vi "optimum.vi"() -> ()   [LabVIEW 2020]
uses:
  <vilib>/MakerHub/LINX/Public/Peripherals/Digital/Digital Read 1 Chan.vi
  <vilib>/MakerHub/LINX/Public/Peripherals/PWM/PWM Set Duty Cycle 1 Chan.vi
  <vilib>/MakerHub/LINX/Public/Peripherals/Digital/Digital Read N Chans.vi
  <vilib>/MakerHub/LINX/Private/Local IO/LinxDigitalRead.vi
  <vilib>/MakerHub/LINX/Public/Utilities/Check Channel.vi
  <vilib>/MakerHub/LINX/Public/Utilities/Open Serial.vi
  <vilib>/MakerHub/LINX/Private/Utilties/Generate Error.vi
  <vilib>/MakerHub/LINX/Public/Peripherals/PWM/PWM Set Duty Cycle N Chans.vi
  <vilib>/MakerHub/LINX/LMH-LINX.lvlib
panel:
  in  "stop":bool
  in  "Serial Port":refnum<visa-resource-name>="N/A"
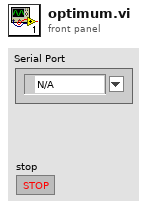
[diagram p1: front panel]
types:
  T1 = typedef "LMH-LINX.lvlib/LINX Ref.ctl" = cluster{"IO":T2, "Interface":T3, "LINX Device Config":T4}
  T2 = typedef "LMH-LINX.lvlib/Platform.ctl" = enum16{"Remote", "Local"}
  T3 = typedef "LMH-LINX.lvlib/Interface.ctl" = enum16{"Serial", "TCP"}
  T4 = typedef "LMH-LINX.lvlib/Device.lvlib/LINX Device Config.ctl" = cluster{"Interface":T3, "COM Port":refnum<visa-resource-name>, "TCP Configuration":T5, "Device Family":u8, "Device ID":u8, "Device Name":string, "TCP Ref":refnum<k5>, "Channels":T6}
  T5 = typedef "LMH-LINX.lvlib/Device.lvlib/TCP Config.ctl" = cluster{"IP Address":string, "Port":u16}
  T6 = typedef "LMH-LINX.lvlib/Channels.ctl" = cluster{"DI":u8[], "DO":u8[], "AI":u8[], "AO":u8[], "PWM":u8[], "QE":u8[], "UART":u8[], "I2C 2":u8[], "SPI":u8[], "CAN":u8[], "Servo":u8[], "AI Ref (V)":dbl, "AI Resolution (Bits)":u8, "AO Ref (V)":dbl, "AO Resolution (Bits)":u8}
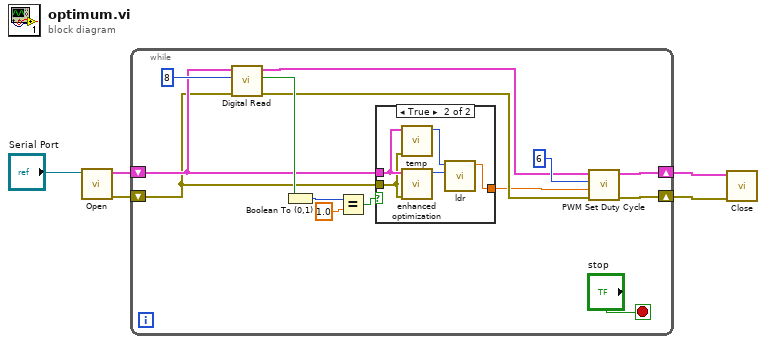
[diagram p0: block diagram]
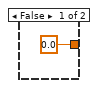
[diagram p2: hidden frame]
diagram:
  n1 = call-poly <vilib>:"Open.vi"("Serial Port"="Serial Port") -> ("Error Out"=w2:errorcluster, "LINX Resource"=w4:T1)  [unwired: 8 in, 1 out]
  n2 = while {
    shift-right: [w18] -> w3
    shift-left: w4 -> [w10]
    shift-right: [w16] -> w1
    shift-left: w2 -> [w9]
    stop <- "stop" stop-if-true
    n3 = call-poly <vilib>:"Digital Read.vi"("Error In"=w9, "DI Channel"=u8 8, "LINX Resource"=w10) -> ("Error Out"=w8:errorcluster, "DI Value"=w15:bool, "LINX Resource"=w11:T1)  [unwired: 6 in]
    n4 = Boolean To (0,1)(Boolean=w15) -> (0, 1=w13:i16)
    n5 = Equal?(x=w13, y=1.0) -> (x = y?=w6:bool)
    n6 = case shown="True" w6 {
      tunnel: w10 -> [_ w25]
      tunnel: w9 -> [_ w24]
      tunnel: [0.0 w23] -> w7
      frame False {
      }
      frame True {
        n7 = call "temp.vi"("error in (no error)"=w24, "LINX Resource"=w25) -> ("Numeric"=w22:i32)  [unwired: 9 in]
        n8 = call "enhanced optimization.vi"("error in (no error)"=w24, "LINX Resource"=w25) -> ("Numeric"=w21:i32)  [unwired: 9 in]
        n9 = call "ldr.vi"("Numeric"=w21, "Numeric 2"=w22) -> ("Numeric 3"=w23:dbl)  [unwired: 9 in]
      }
    }
    n10 = call-poly <vilib>:"PWM Set Duty Cycle.vi"("Error In"=w8, "Duty Cycle (0-1)"=w7, "PWM Channel"=u8 6, "LINX Resource"=w11) -> ("Error Out"=w16:errorcluster, "LINX Resource"=w18:T1)  [unwired: 6 in]
  }
  n11 = call <vilib>:"Close.vi"("Error In"=w1, "LINX Resource"=w3) -> ()  [unwired: 9 in, 1 out]
